vi "PyConv_BlockDiagram.vi"(6 "error in":errorcluster, 9 "PythonConverter_BD in":refnum<class "PyConvBD.lvclass">) -> (0 "error out":errorcluster, 3 "PythonConverter_BD out":refnum<class "PyConvBD.lvclass">, 4 "BlockDiagram":string)   [LabVIEW 2014, in "Raspberry Pi Compatible Compiler for LabVIEW.lvlib" / "PyConvBD.lvclass"]
uses:
  PyConvBD.lvclass
  PyConvBD.lvclass/PyConvBD.ctl
  VI Interpreter/Classes/TopLevelDiagram/TopLevelDiagram.lvclass
  VI Interpreter/Classes/VI Interpreter/VI Interpreter.lvclass
  Parsing/Python Functions.lvlib
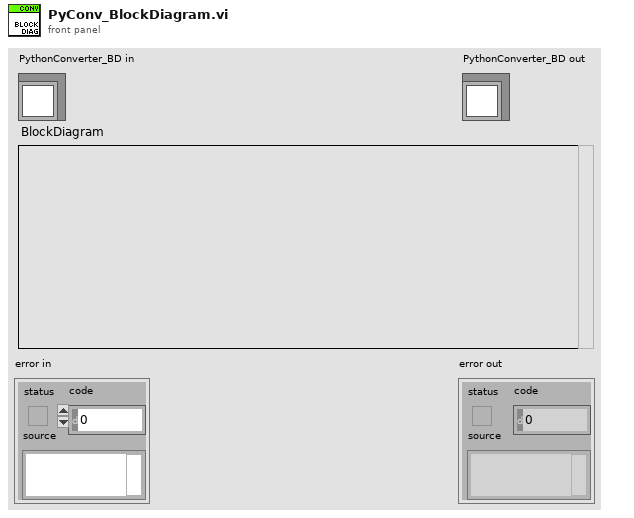
[diagram p1: front panel]
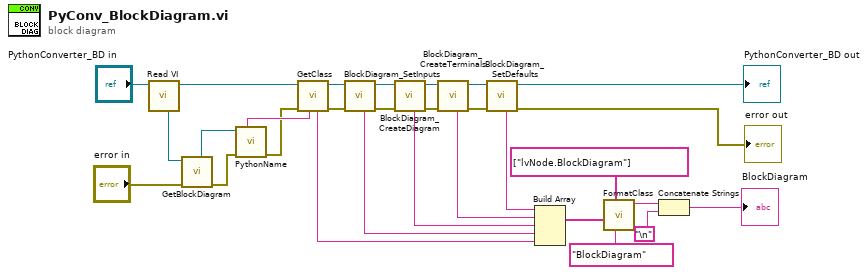
[diagram p0: block diagram]
diagram:
  n1 = call "Read VI.vi"("PythonConverter_BD in"="PythonConverter_BD in") -> ("PythonConverter_BD out"=w24:refnum<class "PyConvBD.lvclass">, "VI Interpreter"=w28:refnum<class "VI Interpreter.lvclass">)  [unwired: 7 in]
  n2 = call "GetBlockDiagram.vi"("error in"="error in", "VI Interpreter in"=w28) -> ("error out"=w25:errorcluster, "TopLevelDiagram"=w26:refnum<class "TopLevelDiagram.lvclass">)  [unwired: 5 in, 1 out]
  n3 = call-dynamic "PythonName.vi"("error in"=w25, "Diagram in"=w26) -> ("error out"=w22:errorcluster, "UID"=w23:string)  [unwired: 6 in, 2 out]
  n4 = call "GetClass.vi"("name"=w23, "error in"=w22, "PythonConverter_BD in"=w24) -> ("error out"=w20:errorcluster, "PythonConverter_BD out"=w21:refnum<class "PyConvBD.lvclass">, "class"=w4:string)  [unwired: 4 in]
  n5 = call "BlockDiagram_SetInputs.vi"("error in"=w20, "PythonConverter_BD in"=w21) -> ("error out"=w18:errorcluster, "PythonConverter_BD out"=w19:refnum<class "PyConvBD.lvclass">, "set_inputs"=w5:string)  [unwired: 5 in]
  n6 = call "BlockDiagram_CreateDiagram.vi"("error in"=w18, "PythonConverter_BD in"=w19) -> ("error out"=w16:errorcluster, "PythonConverter_BD out"=w17:refnum<class "PyConvBD.lvclass">, "create_diagram"=w6:string)  [unwired: 5 in]
  n7 = call "BlockDiagram_CreateTerminals.vi"("error in"=w16, "PythonConverter_BD in"=w17) -> ("error out"=w14:errorcluster, "PythonConverter_BD out"=w15:refnum<class "PyConvBD.lvclass">, "create_terminals"=w7:string)  [unwired: 5 in]
  n8 = call "BlockDiagram_SetDefaults.vi"("error in"=w14, "PythonConverter_BD in"=w15) -> ("error out"=→"error out":errorcluster, "PythonConverter_BD out"=→"PythonConverter_BD out":refnum<class "PyConvBD.lvclass">, "set_defaults"=w8:string)  [unwired: 5 in]
  n9 = Build Array(w8, w7, w6, w5, w4) -> (w11:string[])
  n10 = call "FormatClass.vi"("name"="BlockDiagram", "parameters/ancestors"=string[] ["lvNode.BlockDiagram"], "body"=w11) -> ("python"=w10:string)  [unwired: 8 in]
  n11 = Concatenate Strings(w10, "\n") -> (→"BlockDiagram":string)
